vi "CloseCANBus.vi"(8 "Error In":errorcluster, 11 "Reference In":T1={"VISA resource name"="", "MotorType"=enum."AK80-64", "CAN ID"=1}) -> (0 "Error Out":errorcluster)   [LabVIEW 2019, in "CubeMarsBLDClib.lvlib"]
uses:
  CubeMarsBLDClib.lvlib
  Reference.ctl
  MotorType.ctl
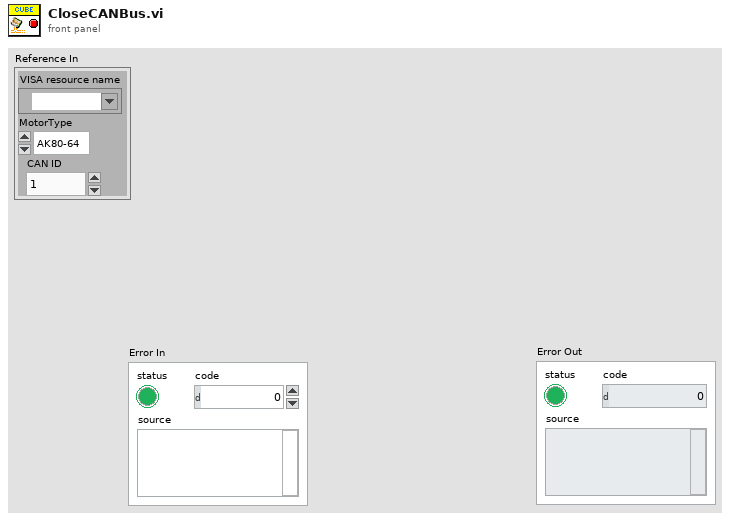
[diagram p1: front panel]
types:
  T1 = typedef "CubeMarsBLDClib.lvlib/Reference.ctl" = cluster{"VISA resource name":refnum<visa-resource-name>, "MotorType":T2, "CAN ID":u32}
  T2 = typedef "CubeMarsBLDClib.lvlib/MotorType.ctl" = enum16{"AK80-64", "AK80-9", "AK80-8", "AK80-6", "AK70-10", "AK60-6", "AK10-9"}
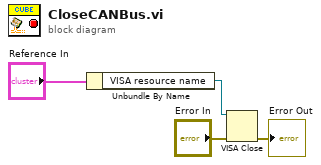
[diagram p0: block diagram]
diagram:
  n1 = Unbundle By Name("Reference In") -> ("VISA resource name"=w1:refnum<visa-resource-name>)
  n2 = VISA Close(VISA resource name=w1, error in (no error)="Error In") -> (error out=→"Error Out":errorcluster)
